vi "Test Process Error Flow Through.vi"(8 "error in (no error)":errorcluster, 11 "Process Test in":refnum<class "Process Dev Test.lvclass">) -> (0 "error out":errorcluster, 3 "Process Test out":refnum<class "Process Dev Test.lvclass">)   [LabVIEW 2020, in "Process Dev Test.lvclass"]
uses:
  Process Dev Test.lvclass
  C:/Program Files (x86)/National Instruments/LabVIEW 2020/vi.lib/Astemes/LUnit/Test Case.lvclass
  source/Framework/Process/Process.lvclass/Process.ctl
  <vilib>/Astemes/LUnit/Test Case.lvclass/Test Case.ctl
  <vilib>/Astemes/LUnit/LUnit Assertion Result.lvclass/LUnit Assertion Result.ctl
  <vilib>/Astemes/LUnit/LUnit Test Case Result.lvclass/LUnit Test Case Result.ctl
  <vilib>/Astemes/LUnit/LUnit Method Result.lvclass/LUnit Method Result.ctl
  source/Framework/Process/Private/SubVIs/Wait for finish.vi
  source/Framework/Process/Protected/Messaging/Enqueue Message.vi
  source/Framework/Process/Private/SubVIs/Set Lifecycle State.vi
  source/Framework/Process/Public/Lifecycle/Get Lifecycle State.vi
  <vilib>/Astemes/LUnit/Set Assertion Type.vi
  <vilib>/Astemes/LUnit/Palette/Pass.vi
  <vilib>/Astemes/LUnit/Palette/Fail.vi
  <vilib>/Astemes/LUnit/Palette/Pass If Equal.vi/cbf50e99-f124-4847-863a-8e9794d3dede.vi
  source/Framework/Process/Private/SubVIs/Handle Debug Data.vi
  <vilib>/Utility/error.llb/Clear Errors.vi
  <vilib>/Astemes/LUnit/LUnit Write Assertion Type.vi
  <vilib>/Astemes/LUnit/Add test result.vi
  <vilib>/Astemes/LUnit/LUnit Write Passed.vi
  <vilib>/Astemes/LUnit/LUnit Write Message.vi
  <vilib>/Astemes/LUnit/LUnit Write Description.vi
  <vilib>/Astemes/LUnit/Compare Variants.vi
  <vilib>/Astemes/LUnit/Describe Comparison.vi
  source/Framework/Logging/Log Debug.vi
  <vilib>/AdvancedString/1D String Array to Delimited String.vi
  <vilib>/Utility/High Resolution Relative Seconds.vi
  <vilib>/Astemes/LUnit/LUnit Record Assertion Result.vi
  <vilib>/Astemes/LUnit/Variant to string.vi
  <vilib>/Astemes/LUnit/LUnit Aggregate Assertion Results.vi
  <vilib>/Astemes/LUnit/Assertion Result/LUnit Read Status.vi
  <vilib>/Astemes/LUnit/LUnit Read Message.vi
  <vilib>/Astemes/LUnit/LUnit Read Description.vi
  <vilib>/Astemes/LUnit/Method Result/LUnit Merge Status.vi
  <vilib>/Astemes/LUnit/LUnit Concatenate result strings.vi
  <vilib>/Utility/error.llb/Error Cluster From Error Code.vi
  source/Framework/Process/Public/Read Name.vi
  <vilib>/Utility/Data Type/Get Type Information.vi
  <vilib>/Utility/LVClass/Get LV Class Name.vi
  <vilib>/ErrorRing/Error Ring.xnode
  <vilib>/Astemes/LUnit/LUnit Assertion Result.lvclass
  source/Framework/Process/Process.lvclass
  <vilib>/Astemes/LUnit/Test Case.lvclass
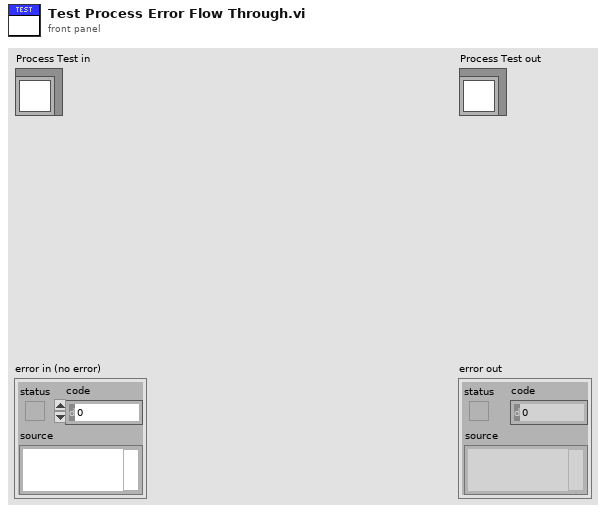
[diagram p1: front panel]
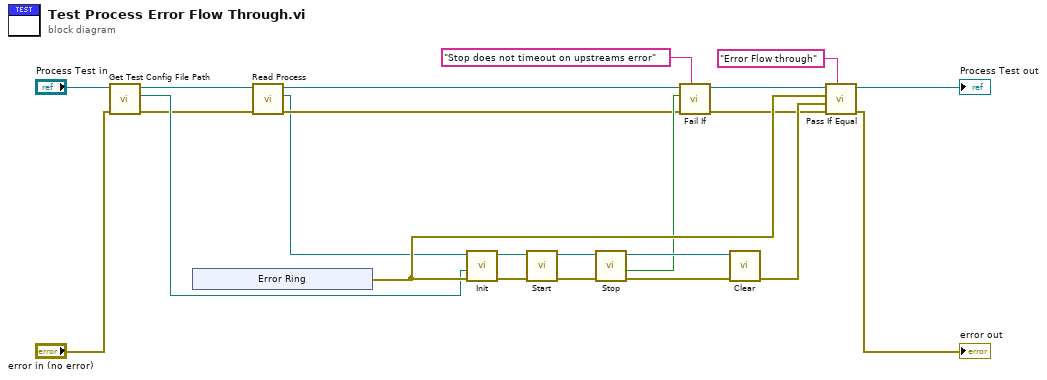
[diagram p0: block diagram]
diagram:
  n1 = call "Get Test Config File Path.vi"("error in (no error)"="error in (no error)", "Process Test In"="Process Test in") -> ("error out"=w5:errorcluster, "Test config path"=w11:path, "Process Test Out"=w3:refnum<class "Process Dev Test.lvclass">)  [unwired: 7 in]
  n2 = xnode "Error Ring"() -> ("error out"=w13:errorcluster)
  n3 = call "Read Process.vi"("error in (no error)"=w5, "Process Test in"=w3) -> ("error out"=w4:errorcluster, "Process.lvclass"=w1:refnum<class "Process.lvclass">, "Process Test out"=w2:refnum<class "Process Dev Test.lvclass">)  [unwired: 7 in]
  n4 = call-dynamic "Init.vi"("error in (no error)"=w13, "Config File Path"=w11, "Process In"=w1) -> ("error out"=w12:errorcluster, "Process Out"=w16:refnum<class "Process.lvclass">)  [unwired: 7 in]
  n5 = call "Start.vi"("error in (no error)"=w12, "Process In"=w16) -> ("error out"=w22:errorcluster, "Process Out"=w23:refnum<class "Process.lvclass">)  [unwired: 7 in, 1 out]
  n6 = call "Stop.vi"("error in (no error)"=w22, "Process In"=w23) -> ("error out"=w18:errorcluster, "timed out?"=w7:bool, "Process Out"=w14:refnum<class "Process.lvclass">)  [unwired: 7 in]
  n7 = call <vilib>:"Fail If.vi"("Description"="Stop does not timeout on upstreams error", "error in (no error)"=w4, "Fail?"=w7, "LUnit Test Case In"=w2) -> ("error out"=w8:errorcluster, "LUnit Test Case Out"=w9:refnum<class "Process Dev Test.lvclass">)  [unwired: 6 in]
  n8 = call-dynamic "Clear.vi"("error in (no error)"=w18, "Process In"=w14) -> ("error out"=w15:errorcluster)  [unwired: 9 in]
  n9 = call <vilib>:"Pass If Equal.vi"("Description"="Error Flow through", "error in (no error)"=w8, "Actual"=w15, "Expected"=w13, "LUnit Test Case In"=w9) -> ("error out"=→"error out":errorcluster, "LUnit Test Case Out"=→"Process Test out":refnum<class "Process Dev Test.lvclass">)  [unwired: 5 in]
